vi "SPI Block Write Bytes.vi"(5 "IntervalTimeUs":i32, 6 "BlockNum":i32, 7 "BlockSize":i32, 9 "pWriteData":u8[](array[numeric])=array[4097 elements], 10 "SPIIndex":i32, 11 "DevHandle":i32) -> (1 "pWriteData out":u8[](array[numeric]), 3 "function return":i32)   [LabVIEW 2010, in "usb2spi.lvlib"]
doc: "int WINAPI SPI_BlockWriteBytes(int DevHandle,int SPIIndex,unsigned char *pWriteData,int BlockSize,int BlockNum,int IntervalTimeUs);"
uses:
  usb2spi.lvlib
  USB2XXX/trunk/USB2XXX/USB2XXX/vs2010/Release/USB2XXX.dll
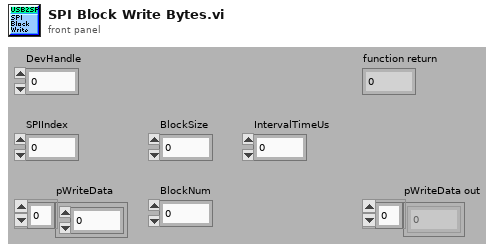
[diagram p1: front panel]
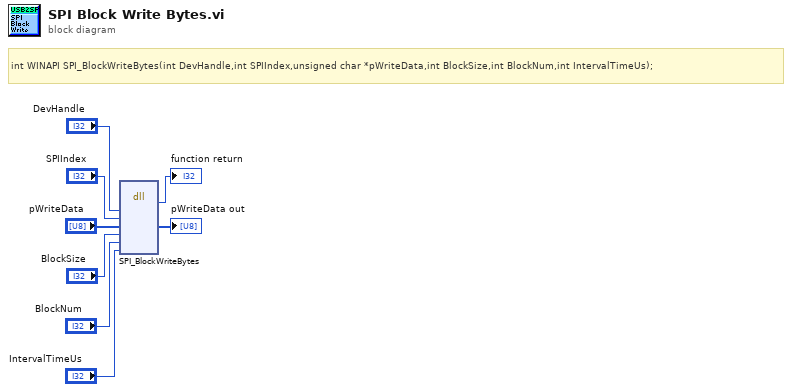
[diagram p0: block diagram]
diagram:
  # "int WINAPI SPI_BlockWriteBytes(int DevHandle,int SPIIndex,unsigned char *pWriteData,int BlockSize,int BlockNum,int IntervalTimeUs);"
  n1 = dll-call lib="E:/OtherWork/STM32/USB2XXX/trunk/USB2XXX/USB2XXX/vs2010/Release/USB2XXX.*" fn="SPI_BlockWriteBytes"("DevHandle"="DevHandle", "SPIIndex"="SPIIndex", "pWriteData"="pWriteData", "BlockSize"="BlockSize", "BlockNum"="BlockNum", "IntervalTimeUs"="IntervalTimeUs") -> (→"function return":i32, "pWriteData"=→"pWriteData out":u8[])  [unwired: 8 in, 2 out]
